vi "IntMsgSetTcpDvr.vi"() -> (1 "message name":string)   [LabVIEW 2017, in "ServerComm.lvlib"]
uses:
  <vilib>/addons/InsightCM/Devices/Shared/Common/ServerComm/ServerComm.lvlib
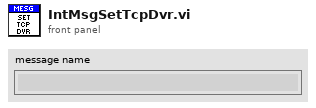
[diagram p1: front panel]
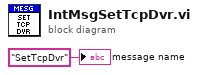
[diagram p0: block diagram]
diagram:
  "message name" <- "SetTcpDvr" ("ProcessName")
